vi "Untitled 2.vi"() -> ()   [LabVIEW 2018]
uses:
  <instrlib>/Thorlabs_FW102C/Thorlabs_FW102C.lvlib
panel:
  out "Connected? 3":bool
  out "Connected? 2":bool
  out "Connected?":bool
  in  "Stop":bool
  out "NDFW102C out":i32
  in  "NDFW Serial Port":string="COM5"
  out "RFW102C out":i32=1
  in  "RFW Serial Port":string="COM3"
  out "error out":errorcluster
  out "TFW102C out":i32
  in  "TFW Serial Port":string="COM4"
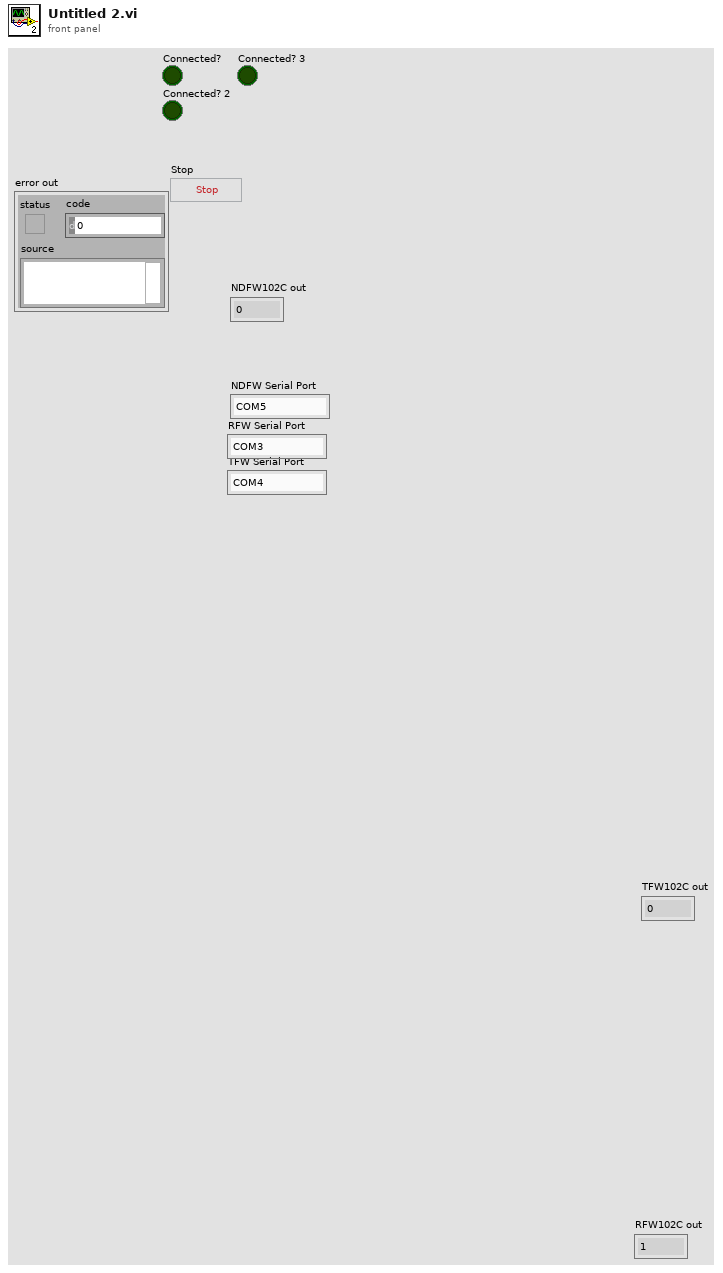
[diagram p1: front panel]
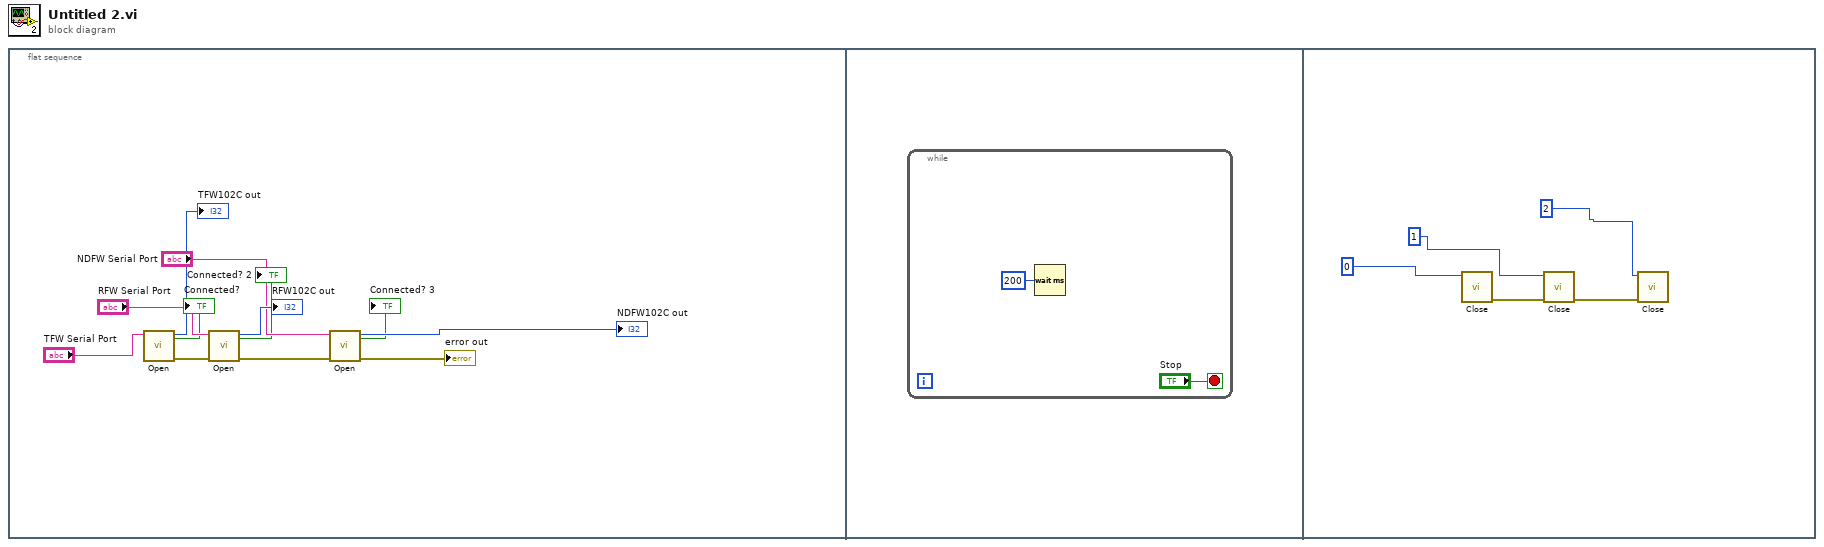
[diagram p0: block diagram]
diagram:
  n1 = flat-sequence {
    frame #0 {
      n2 = call <instrlib>:"Open.vi"("Serial Port"="TFW Serial Port") -> ("error out"=w10:errorcluster, "FW102C out"=→"TFW102C out":i32, "Connected?"=→"Connected?":bool)  [unwired: 8 in]
      n3 = call <instrlib>:"Open.vi"("error in (no error)"=w10, "Serial Port"="RFW Serial Port") -> ("error out"=w11:errorcluster, "FW102C out"=→"RFW102C out":i32, "Connected?"=→"Connected? 2":bool)  [unwired: 7 in]
      n4 = call <instrlib>:"Open.vi"("error in (no error)"=w11, "Serial Port"="NDFW Serial Port") -> ("error out"=→"error out":errorcluster, "FW102C out"=→"NDFW102C out":i32, "Connected?"=→"Connected? 3":bool)  [unwired: 7 in]
    }
    frame #1 {
      n5 = while {
        stop <- "Stop" stop-if-true
        n6 = Wait (ms)(milliseconds to wait=u32 200) -> ()  [unwired: 1 out]
      }
    }
    frame #2 {
      n7 = call <instrlib>:"Close.vi"("FW102C in"=0) -> ("error out"=w19:errorcluster)  [unwired: 10 in]
      n8 = call <instrlib>:"Close.vi"("error in (no error)"=w19, "FW102C in"=1) -> ("error out"=w18:errorcluster)  [unwired: 9 in]
      n9 = call <instrlib>:"Close.vi"("error in (no error)"=w18, "FW102C in"=2) -> ()  [unwired: 9 in, 1 out]
    }
  }
